vi "Ref_Num_Generate_Report_NEW.vi"(0 "LowCapMode?":refnum<vi>, 1 "Test Part":refnum<vi>, 2 "Test Voltages(V)":refnum<vi>, 3 "T.V. True":refnum<vi>, 4 "Stop":refnum<vi>, 5 "error in (no error)":errorcluster, 6 "Array":refnum<vi>, 7 "Chart Voltage Generation Method":refnum<vi>, 8 "XY Graph NEW":refnum<vi>, 10 "CapTest?":refnum<vi>, 11 "Polarity for Max Voltage":refnum<vi>, 12 "Test Voltages Chosen":refnum<vi>, 13 "Capacitance(pF)":refnum<vi>, 14 "Min Voltage":refnum<vi>, 15 "Max Voltage":refnum<vi>, 17 "Status : Running":refnum<vi>, 18 "Next Part":refnum<vi>) -> (19 "error out":errorcluster)   [LabVIEW 2020]
uses:
  Global 1.vi
  <vilib>/Utility/file.llb/Write Delimited Spreadsheet (DBL).vi
  <vilib>/Utility/file.llb/Write Delimited Spreadsheet (string).vi
panel:
  out "error out 2":errorcluster
  in  "Test Voltages TRUE":bool
  in  "Test Voltages Results Temp Array":dbl[](array[numeric]) format="%_6g"
  out "Status : Running+-":bool
  in  "Test Voltages (in)":dbl[](array[numeric])=[0.0, 0.1, 0.2, 0.3, 0.4, 0.5, 0.7, 1.0, 2.0, 3.0, 4.0, 5.0, 7.0, 10.0, 20.0, 30.0, 40.0, 50.0, 70.0, 100.0, 200.0]
  in  "Capacitance Results Temp Array":dbl[](array[numeric]) format="%_10g"
  in  "Default":i32=1
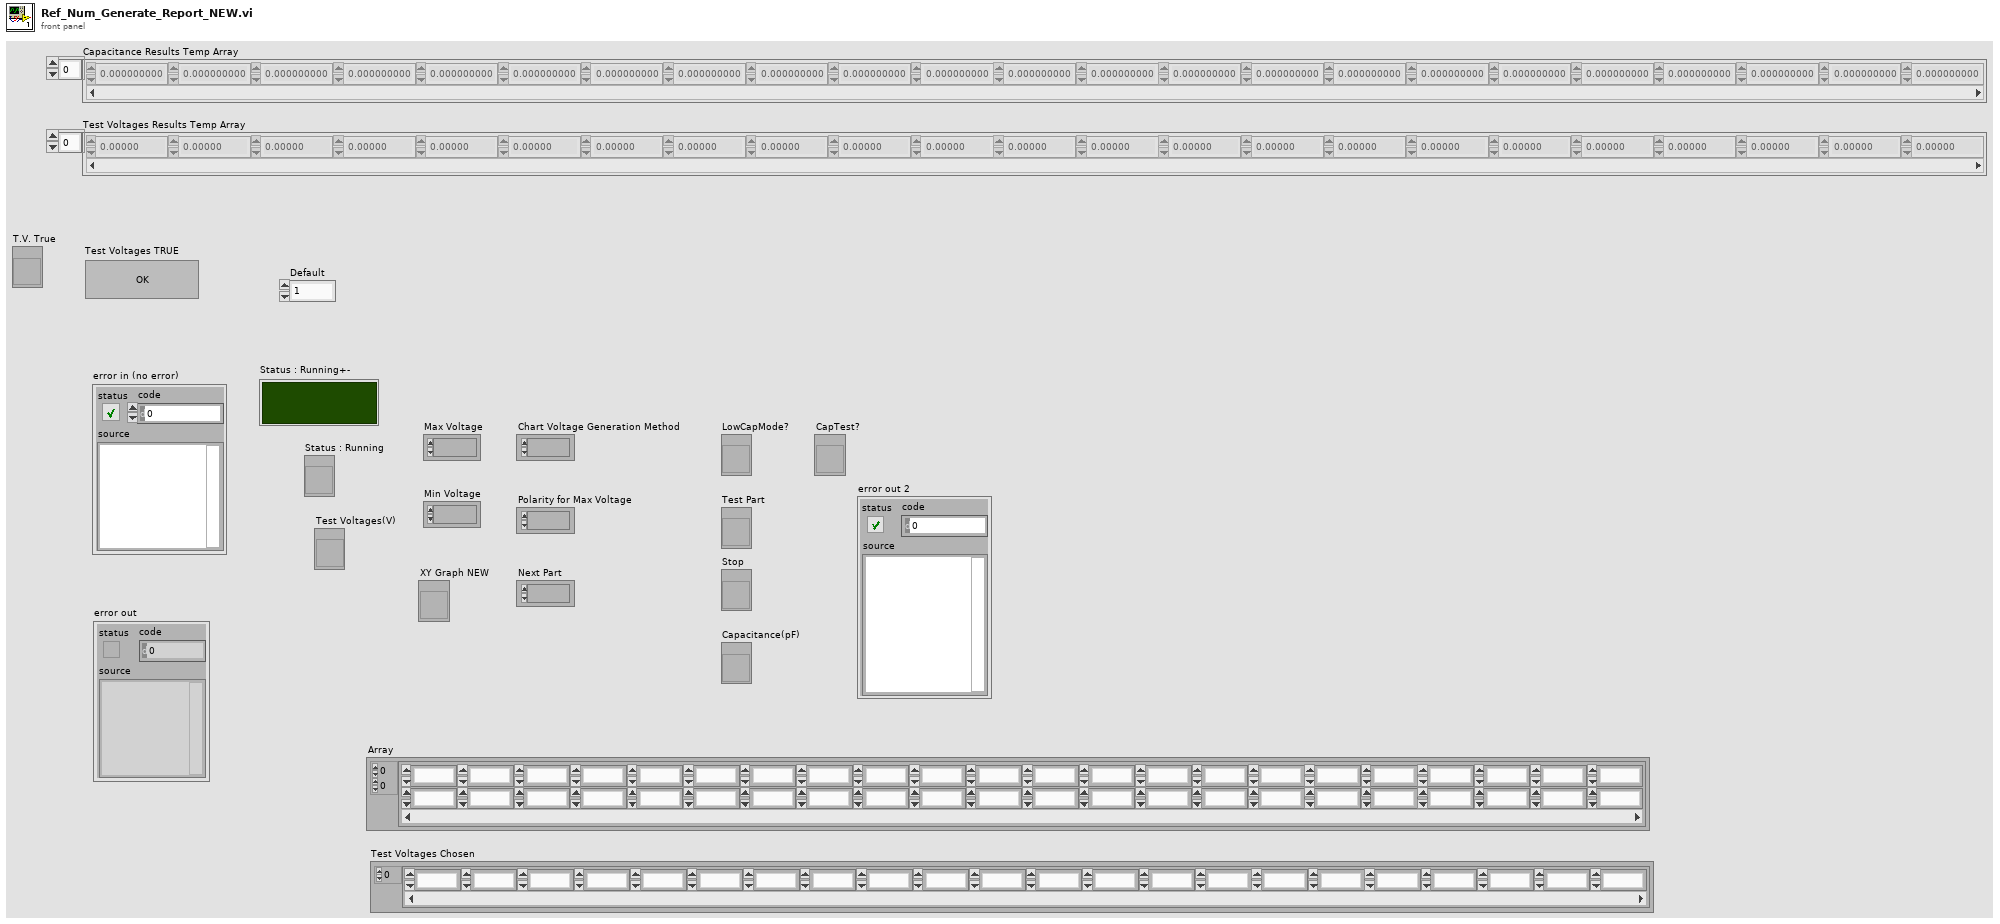
[diagram p1: front panel]
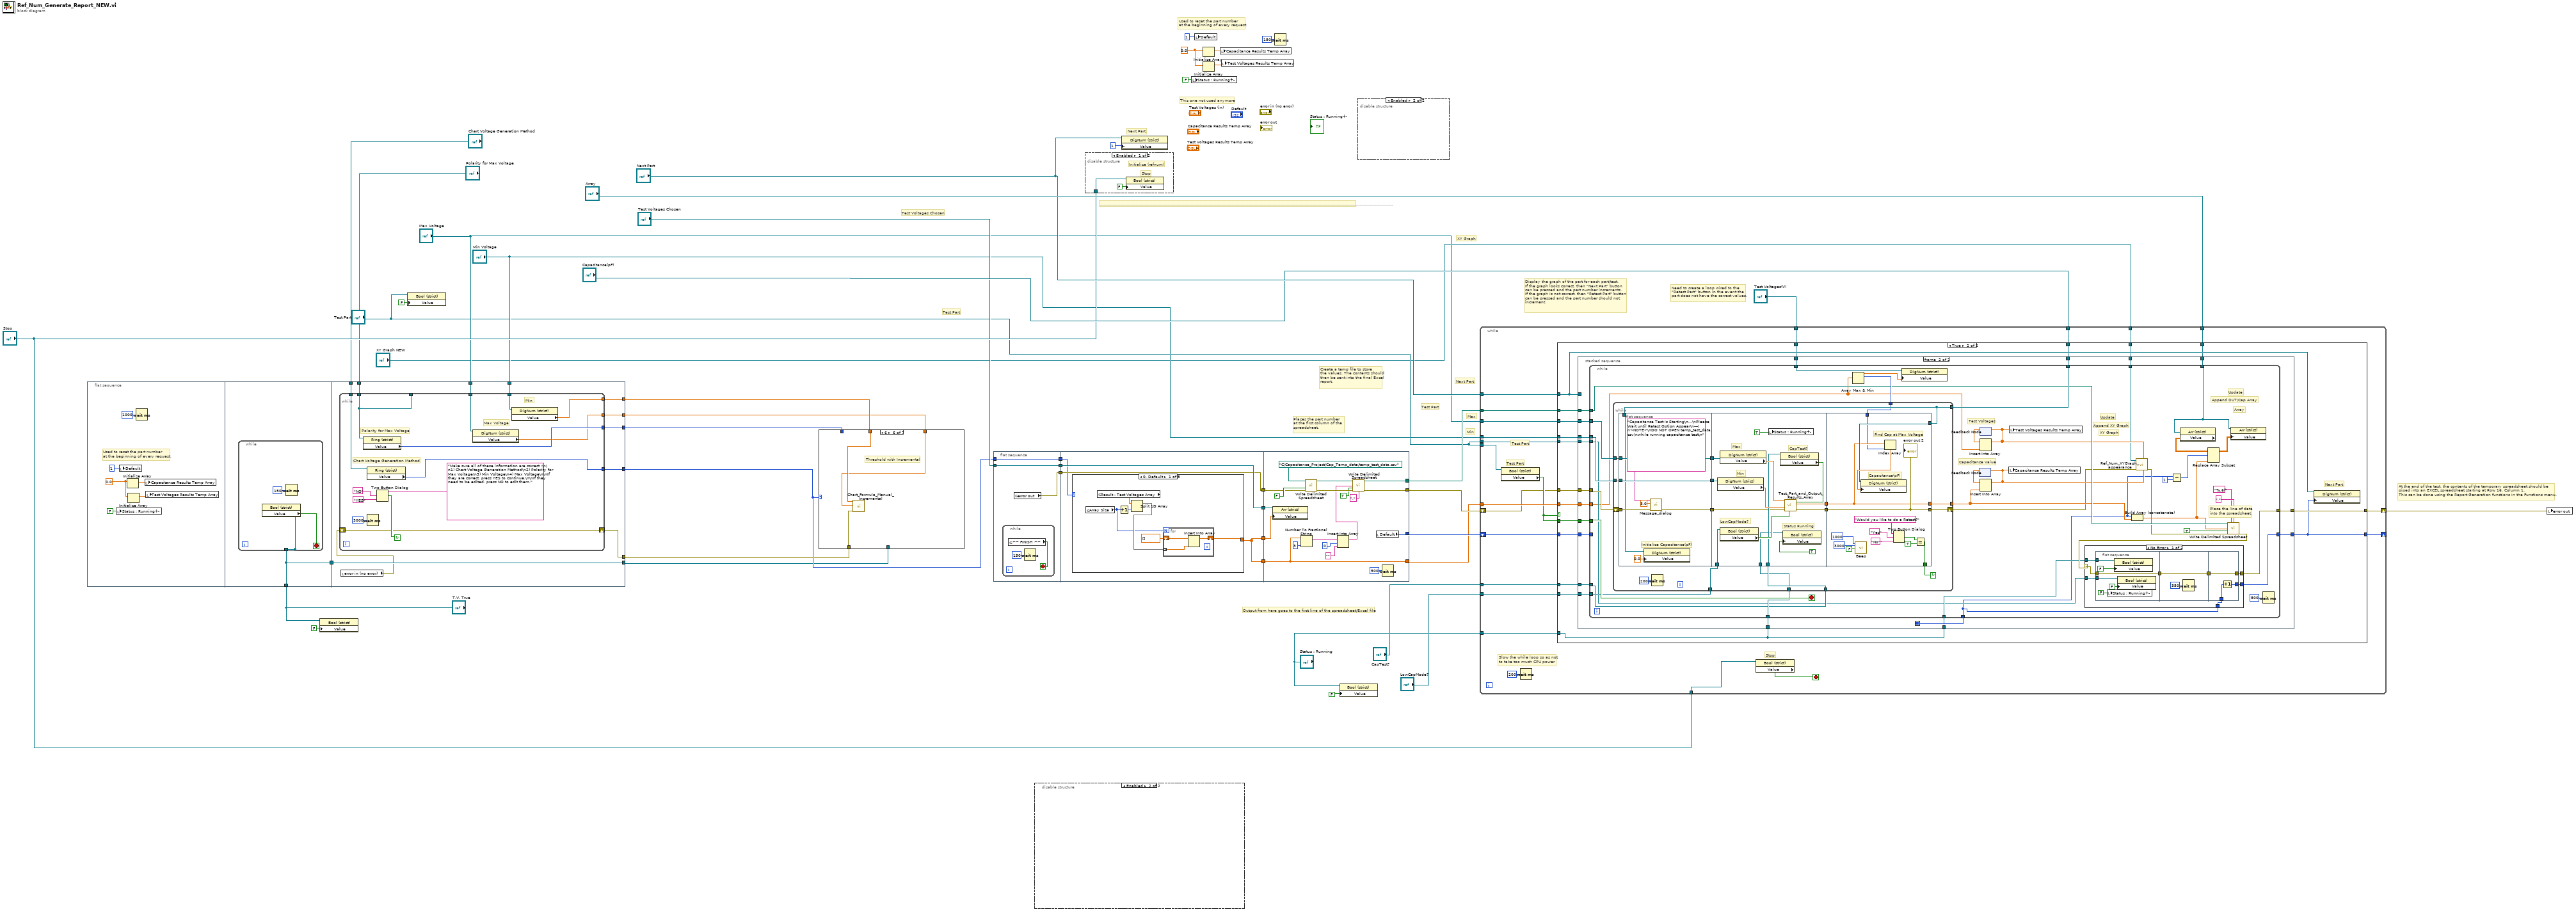
[diagram p0: block diagram]
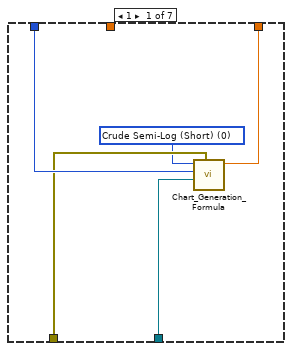
[diagram p2: hidden frame]
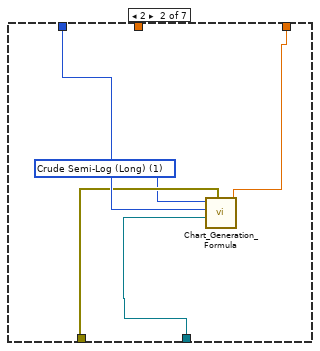
[diagram p3: hidden frame]
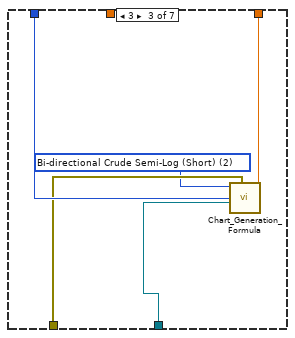
[diagram p4: hidden frame]
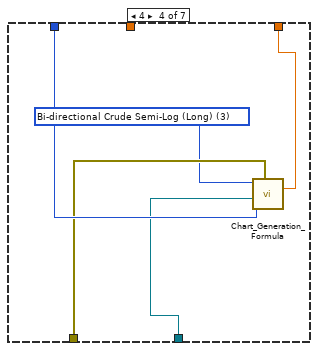
[diagram p5: hidden frame]
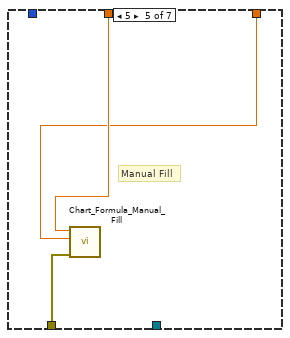
[diagram p6: hidden frame]
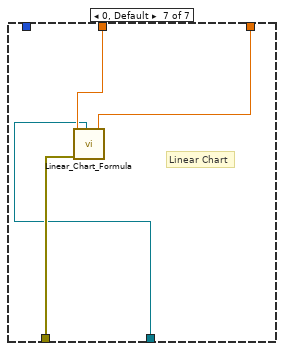
[diagram p7: hidden frame]
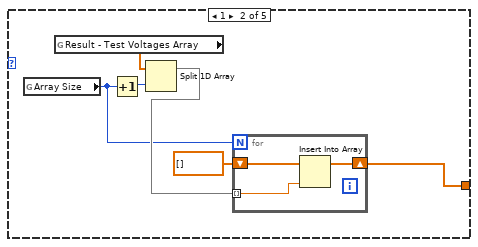
[diagram p8: hidden frame]
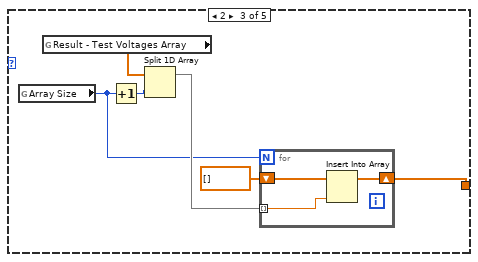
[diagram p9: hidden frame]
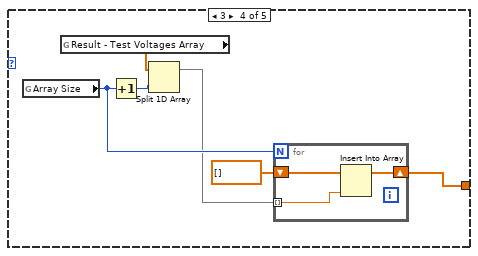
[diagram p10: hidden frame]
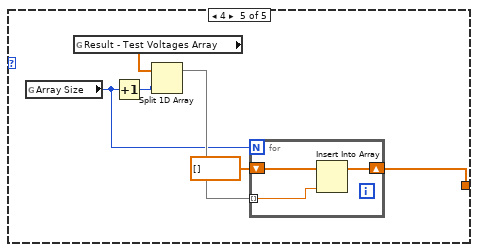
[diagram p11: hidden frame]
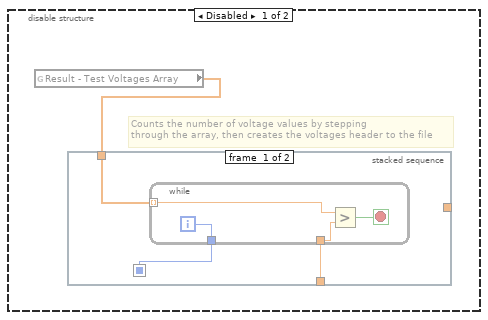
[diagram p13: hidden frame]
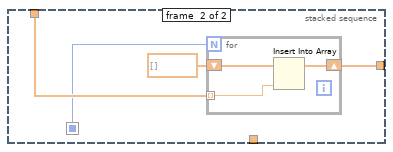
[diagram p14: hidden frame]
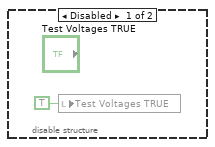
[diagram p15: hidden frame]
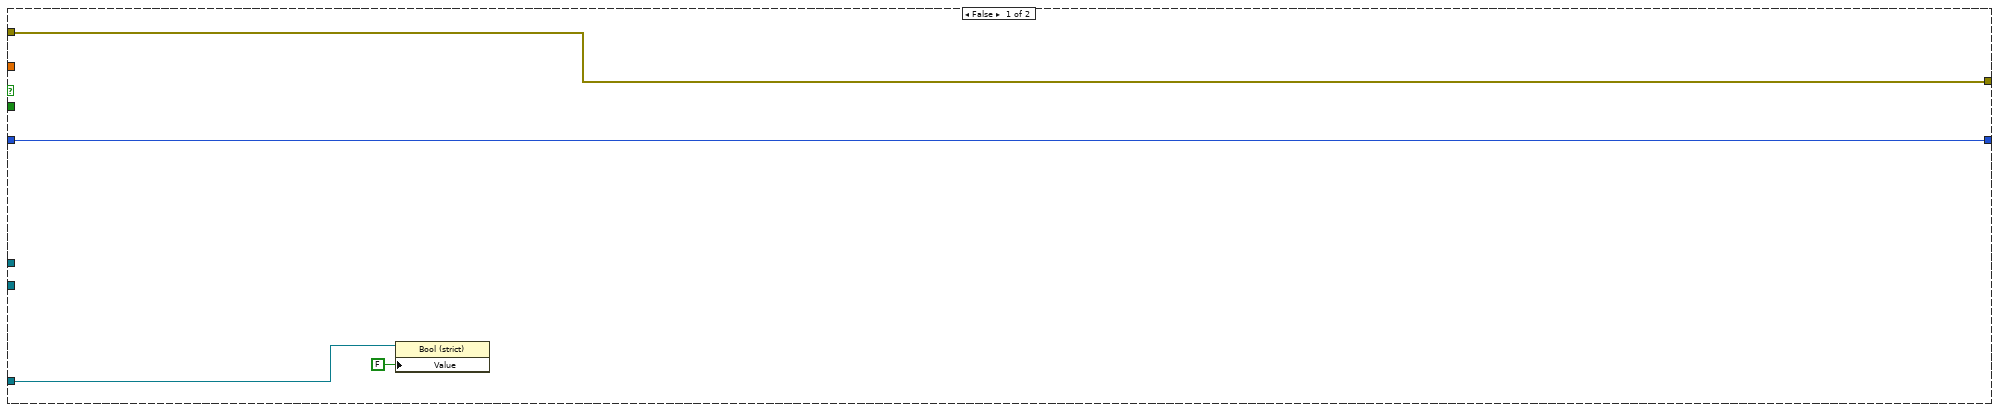
[diagram p16: hidden frame]
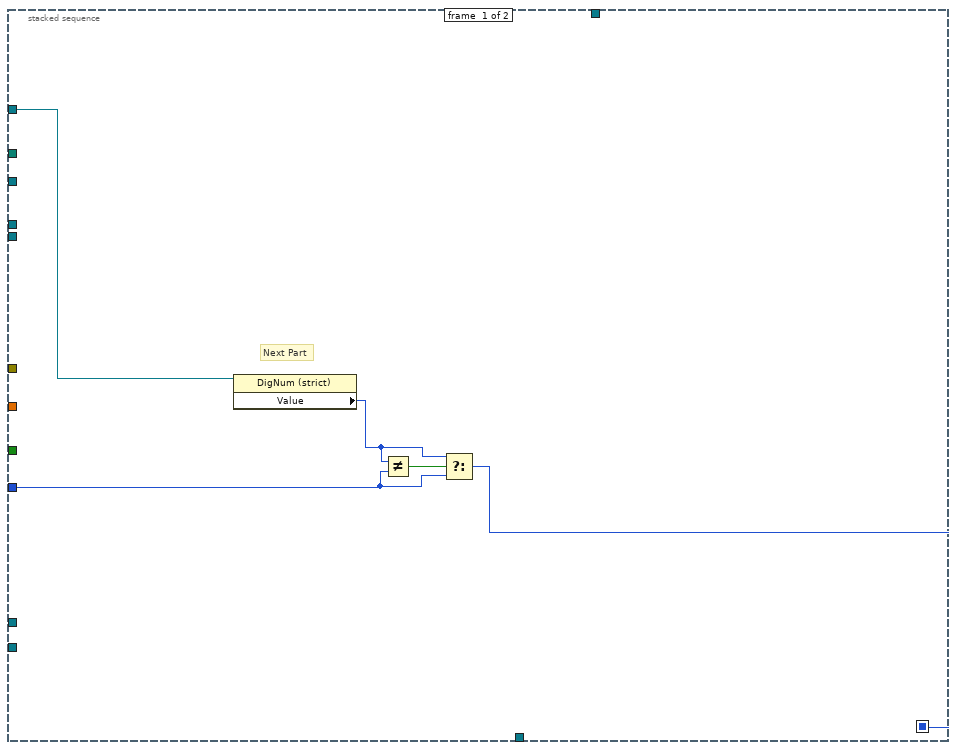
[diagram p17: hidden frame]
diagram:
  w6 = 0.0 ("element")
  # "Places the part number\nat the first column of the \nspreadsheet."
  # "Used to reset the part number\nat the beginning of every request."
  # "XY Graph"
  # "Need to create a loop wired to the \n\"Retest Part\" button in the event the \npart does not have the correct values."
  # "Display the graph of the part for each part/test.\nIf the graph looks correct, then \"Next Part\" button\ncan be pressed and the part number increments.\nIf the graph is not correct, then \"Retest Part\" button\ncan be pressed and the part number should not\nincrement."
  # "This one not used anymore"
  # "Test Part"
  # "Test Part"
  # "Min"
  # "Max"
  # "Test Voltages Chosen"
  # "....................................................................................................................................................................................................................................."
  # "Next Part"
  # "Next Part"
  # "At the end of the test, the contents of the temporary spreadsheet should be\npiped into an EXCEL spreadsheet starting at Row 16, Column 1. \nThis can be done using the Report Generation functions in the Functions menu."
  # "Create a temp file to store\nthe values. The contents should\nthen be sent into the final Excel\nreport."
  # "Output from here goes to the first line of the spreadsheet/Excel file"
  n1 = flat-sequence {
    tunnel: "T.V. True" -> [w52]
    tunnel: [w52] -> w1
    tunnel: "Chart Voltage Generation Method" -> [w66]
    tunnel: "Polarity for Max Voltage" -> [w65]
    tunnel: "Max Voltage" -> [w64]
    tunnel: "Min Voltage" -> [w63]
    tunnel: w1 -> [w58]
    tunnel: [w62] -> w21
    tunnel: [w61] -> w20
    tunnel: [w60] -> w19
    tunnel: [w59] -> w18
    tunnel: [w56] -> w17
    tunnel: [w58] -> w2
    frame #0 {
      w48 = 0.0 ("element")
      # "Used to reset the part number\nat the beginning of every request."
      n2 = local write "Status : Running+-"(FALSE ("Status : Running+-")) -> ()
      n3 = local write "Default"(1 ("New Part Number")) -> ()
      n4 = Initialize Array(w48) -> (w49:dbl[])  [unwired: 1 in]
      n5 = Initialize Array(w48) -> (w50:dbl[])  [unwired: 1 in]
      n6 = Wait (ms)(milliseconds to wait=u32 1000) -> ()  [unwired: 1 out]
      n7 = local write "Capacitance Results Temp Array"(w49) -> ()
      n8 = local write "Test Voltages Results Temp Array"(w50) -> ()
    }
    frame #1 {
      n9 = while {
        tunnel: w52 -> [w54]
        tunnel: [w54] -> _
        stop <- w55 stop-if-true
        n10 = property class="Bool (strict)"(reference=w54) -> ("Value"=w55:bool)  [unwired: 1 in, 2 out]
        n11 = Wait (ms)(milliseconds to wait=u32 150) -> ()  [unwired: 1 out]
      }
    }
    frame #2 {
      n12 = local read "error in (no error)"() -> (w57:errorcluster)
      n13 = while {
        tunnel: w66 -> [w75]
        tunnel: [w74] -> w59
        tunnel: w65 -> [w68]
        tunnel: [w73] -> w60
        tunnel: w64 -> [w72]
        tunnel: [w71] -> w61
        tunnel: w63 -> [w70]
        tunnel: [w69] -> w62
        tunnel: [w68] -> _
        shift-right: [w67] -> w56
        shift-left: w57 -> [w67]
        stop <- w77 continue-if-true
        # "Min"
        # "Max Voltage"
        # "Polarity for Max Voltage"
        # "Chart Voltage Generation Method"
        n14 = property class="Ring (strict)"(reference=w68) -> ("Value"=w73:u16)  [unwired: 1 in, 2 out]
        n15 = Wait (ms)(milliseconds to wait=u32 3000) -> ()  [unwired: 1 out]
        n16 = property class="Ring (strict)"(reference=w75) -> ("Value"=w74:u16)  [unwired: 1 in, 2 out]
        n17 = Two Button Dialog(message="Make sure all of these information are correct :\n\n1) Chart Voltage Generation Method\n2) Polarity for Max Voltage\n3) Min Voltage\n4) Max Voltage\n\nIf they are correct, press YES to continue.\n\nIf they need to be edited, press NO to edit them.", 1:"YES" ("Right Button Text (\"Cancel\")"), 2:"NO" ("Left Button Text (\"Yes\")")) -> (T button?=w77:bool)
        n18 = property class="DigNum (strict)"(reference=w72) -> ("Value"=w71:dbl)  [unwired: 1 in, 2 out]
        n19 = property class="DigNum (strict)"(reference=w70) -> ("Value"=w69:dbl)  [unwired: 1 in, 2 out]
      }
    }
  }
  n20 = property class="Bool (strict)"(reference="T.V. True", "Value"=FALSE) -> ()  [unwired: 1 in, 2 out]
  n21 = property class="Bool (strict)"(reference="Test Part", "Value"=FALSE) -> ()  [unwired: 1 in, 2 out]
  n22 = case shown="6" w18 {
    tunnel: w19 -> [w85 w90 w95 w100 _ _ _]
    tunnel: w20 -> [w84 w89 w94 w99 w101 w104 w109]
    tunnel: w2 -> [w83 w88 w93 w98 _ _ w107]
    tunnel: w17 -> [w82 w87 w92 w97 w103 w106 w110]
    tunnel: w21 -> [_ _ _ _ w102 w105 w108]
    frame 1 {
      w81 = u16 0 items=[" Crude Semi-Log (Short)", "Crude Semi-Log (Long)", "Bi-directional Crude Semi-Log (Short)", "Bi-directional Crude Semi-Log (Long)"] ("Type of Chart")
      n23 = call "Chart_Generation_Formula.vi"("Max Voltage"=w84, "error in (no error)"=w82, "CGF_Input"=w83, "Polarity for Max Voltage"=w85, "Type of Chart"=w81) -> ()  [unwired: 4 in, 3 out]
    }
    frame 2 {
      w86 = u16 1 items=[" Crude Semi-Log (Short)", "Crude Semi-Log (Long)", "Bi-directional Crude Semi-Log (Short)", "Bi-directional Crude Semi-Log (Long)"] ("Type of Chart")
      n24 = call "Chart_Generation_Formula.vi"("Max Voltage"=w89, "error in (no error)"=w87, "CGF_Input"=w88, "Polarity for Max Voltage"=w90, "Type of Chart"=w86) -> ()  [unwired: 4 in, 3 out]
    }
    frame 3 {
      w91 = u16 2 items=[" Crude Semi-Log (Short)", "Crude Semi-Log (Long)", "Bi-directional Crude Semi-Log (Short)", "Bi-directional Crude Semi-Log (Long)"] ("Type of Chart")
      n25 = call "Chart_Generation_Formula.vi"("Max Voltage"=w94, "error in (no error)"=w92, "CGF_Input"=w93, "Polarity for Max Voltage"=w95, "Type of Chart"=w91) -> ()  [unwired: 4 in, 3 out]
    }
    frame 4 {
      w96 = u16 3 items=[" Crude Semi-Log (Short)", "Crude Semi-Log (Long)", "Bi-directional Crude Semi-Log (Short)", "Bi-directional Crude Semi-Log (Long)"] ("Type of Chart")
      n26 = call "Chart_Generation_Formula.vi"("Max Voltage"=w99, "error in (no error)"=w97, "CGF_Input"=w98, "Polarity for Max Voltage"=w100, "Type of Chart"=w96) -> ()  [unwired: 4 in, 3 out]
    }
    frame 5 {
      # "Manual Fill"
      n27 = call "Chart_Formula_Manual_Fill.vi"("error in (no error)"=w103, "Max Voltage"=w101, "Min Voltage"=w102) -> ()  [unwired: 9 in]
    }
    frame 6 {
      # "Threshold with Incremental"
      n28 = call "Chart_Formula_Manual_Incremental.vi"("error in (no error)"=w106, "Max Voltage"=w104, "Min Voltage"=w105) -> ()  [unwired: 8 in]
    }
    frame 0, Default {
      # "Linear Chart"
      n29 = call "Linear_Chart_Formula.vi"("Max Voltage"=w109, "Start"=w107, "error in (no error)"=w110, "Min Voltage"=w108) -> ()  [unwired: 7 in, 1 out]
    }
  }
  n30 = flat-sequence {
    tunnel: w18 -> [w112]
    tunnel: "Test Voltages Chosen" -> [w113]
    tunnel: [w113] -> w25
    tunnel: [w112] -> w24
    tunnel: [w111] -> w22
    tunnel: [w118] -> w30
    tunnel: [w116] -> w29
    tunnel: [w119] -> w28
    tunnel: [w118] -> w27
    tunnel: w25 -> [w119]
    tunnel: w24 -> [w117]
    tunnel: w22 -> [w116]
    tunnel: w30 -> [w166]
    tunnel: w29 -> [w169]
    tunnel: w28 -> [w168]
    tunnel: w27 -> [w167]
    tunnel: [w179] -> w45
    tunnel: [w176] -> w44
    tunnel: [w174] -> w35
    tunnel: [w166] -> w26
    frame #0 {
      n31 = while {
        stop <- w115 stop-if-true
        n32 = global read "Global 1.vi" "~~ FINISH ~~"() -> (w115:bool)
        n33 = Wait (ms)(milliseconds to wait=u32 150) -> ()  [unwired: 1 out]
      }
      n34 = global read "Global 1.vi" "error out"() -> (w111:errorcluster)
    }
    frame #1 {
      n35 = case shown="0, Default" w117 {
        tunnel: [w120 w129 w138 w147 w156] -> w118
        frame 0, Default {
          n36 = global read "Global 1.vi" "Array Size"() -> (w122:i32)
          n37 = global read "Global 1.vi" "Result - Test Voltages Array"() -> (w125:dbl[])
          n38 = Increment(x=w122) -> (x+1=w124:i32)
          n39 = Split 1D Array(array=w125, index=w124) -> (first subarray=w123:dbl[])  [unwired: 1 out]
          n40 = for {
            N: w122 -> [_]
            tunnel: w123 -> [w128] mode=indexing
            shift-right: [w126] -> w120
            shift-left: dbl[] [] -> [w127]
            n41 = Insert Into Array(array=w127, new element=w128) -> (w126:dbl[])  [unwired: 1 in]
          }
        }
        frame 1 {
          n42 = global read "Global 1.vi" "Array Size"() -> (w130:i32)
          n43 = global read "Global 1.vi" "Result - Test Voltages Array"() -> (w134:dbl[])
          n44 = Increment(x=w130) -> (x+1=w133:i32)
          n45 = Split 1D Array(array=w134, index=w133) -> (first subarray=w131:dbl[])  [unwired: 1 out]
          n46 = for {
            N: w130 -> [_]
            tunnel: w131 -> [w137] mode=indexing
            shift-right: [w135] -> w129
            shift-left: dbl[] [] -> [w136]
            n47 = Insert Into Array(array=w136, new element=w137) -> (w135:dbl[])  [unwired: 1 in]
          }
        }
        frame 2 {
          n48 = global read "Global 1.vi" "Array Size"() -> (w139:i32)
          n49 = global read "Global 1.vi" "Result - Test Voltages Array"() -> (w142:dbl[])
          n50 = Increment(x=w139) -> (x+1=w143:i32)
          n51 = Split 1D Array(array=w142, index=w143) -> (first subarray=w140:dbl[])  [unwired: 1 out]
          n52 = for {
            N: w139 -> [_]
            tunnel: w140 -> [w146] mode=indexing
            shift-right: [w144] -> w138
            shift-left: dbl[] [] -> [w145]
            n53 = Insert Into Array(array=w145, new element=w146) -> (w144:dbl[])  [unwired: 1 in]
          }
        }
        frame 3 {
          n54 = global read "Global 1.vi" "Array Size"() -> (w149:i32)
          n55 = global read "Global 1.vi" "Result - Test Voltages Array"() -> (w151:dbl[])
          n56 = Increment(x=w149) -> (x+1=w152:i32)
          n57 = Split 1D Array(array=w151, index=w152) -> (first subarray=w148:dbl[])  [unwired: 1 out]
          n58 = for {
            N: w149 -> [_]
            tunnel: w148 -> [w155] mode=indexing
            shift-right: [w153] -> w147
            shift-left: dbl[] [] -> [w154]
            n59 = Insert Into Array(array=w154, new element=w155) -> (w153:dbl[])  [unwired: 1 in]
          }
        }
        frame 4 {
          n60 = global read "Global 1.vi" "Array Size"() -> (w157:i32)
          n61 = global read "Global 1.vi" "Result - Test Voltages Array"() -> (w160:dbl[])
          n62 = Increment(x=w157) -> (x+1=w161:i32)
          n63 = Split 1D Array(array=w160, index=w161) -> (first subarray=w158:dbl[])  [unwired: 1 out]
          n64 = for {
            N: w157 -> [_]
            tunnel: w158 -> [w164] mode=indexing
            shift-right: [w162] -> w156
            shift-left: dbl[] [] -> [w163]
            n65 = Insert Into Array(array=w163, new element=w164) -> (w162:dbl[])  [unwired: 1 in]
          }
        }
      }
    }
    frame #2 {
      n66 = property class="Arr (strict)"(reference=w168, "Value"=w167) -> ()  [unwired: 1 in, 2 out]
      n67 = Number To Fractional String(number=w166, precision (6)=i16 3) -> (F-format string=w182:string[])  [unwired: 2 in]
      n68 = call-poly <vilib>:"Write Delimited Spreadsheet.vi"("file path (dialog if empty)"=path "C:/Capacitance_Project/Cap_Temp_data/temp_test_data.csv", "append to file? (new file:F)"=FALSE, "error in (no error)"=w169) -> ("new file path (Not A Path if cancelled)"=w177:path, "error out"=w175:errorcluster)  [unwired: 11 in]
      n69 = Insert Into Array(array=w182, index=0, new element="" ("new element/subarray")) -> (w173:string[])
      n70 = call-poly <vilib>:"Write Delimited Spreadsheet.vi"("file path (dialog if empty)"=w177, "1D data"=w173, "append to file? (new file:F)"=TRUE, "error in (no error)"=w175, "delimiter (\\t)"="," ("delimiter (\\t)")) -> ("new file path (Not A Path if cancelled)"=w176:path, "error out"=w174:errorcluster)  [unwired: 9 in]
      n71 = local read "Default"() -> (w179:i32)
      n72 = Wait (ms)(milliseconds to wait=u32 500) -> ()  [unwired: 1 out]
    }
  }
  n73 = disable-structure shown="Enabled" {
    frame Disabled {
      # "Counts the number of voltage values by stepping\nthrough the array, then creates the voltages header to the file"
      n74 = global read "Global 1.vi" "Result - Test Voltages Array"() -> (w184:dbl[])
      n75 = stacked-sequence {
        seq-local: [w186 _] -> [_ w193]
        tunnel: w184 -> [w187 w194]
        tunnel: [_ w195] -> _
        tunnel: _ -> [w185 _]
        frame #0 {
          n76 = while {
            tunnel: w187 -> [w190] mode=indexing
            tunnel: [w189] -> w186
            tunnel: w185 -> [w188]
            i -> [w189]
            stop <- w191 stop-if-true
            n77 = Greater?(x=w190, y=w188) -> (0:w191:bool)
          }
        }
        frame #1 {
          n78 = for {
            N: w193 -> [_]
            tunnel: w194 -> [w198] mode=indexing
            shift-right: [w196] -> w195
            shift-left: dbl[] [] -> [w197]
            n79 = Insert Into Array(array=w197, new element=w198) -> (w196:dbl[])  [unwired: 1 in]
          }
        }
      }
    }
    frame Enabled {
    }
  }
  n80 = disable-structure shown="Enabled" {
    disable-tunnel: "Stop" -> [w199 _]
    frame Enabled {
      # "Stop"
      # "Initialize (refnum)"
      n81 = property class="Bool (strict)"(reference=w199, "Value"=FALSE) -> ()  [unwired: 1 in, 2 out]
    }
    frame Disabled {
    }
  }
  n82 = property class="DigNum (strict)"(reference="Next Part", "Value"=1) -> ()  [unwired: 1 in, 2 out]
  n83 = local write "Status : Running+-"(FALSE ("Status : Running+-")) -> ()
  n84 = local write "Default"(1 ("New Part Number")) -> ()
  n85 = Initialize Array(w6) -> (w5:dbl[])  [unwired: 1 in]
  n86 = Initialize Array(w6) -> (w4:dbl[])  [unwired: 1 in]
  n87 = local write "Capacitance Results Temp Array"(w5) -> ()
  n88 = local write "Test Voltages Results Temp Array"(w4) -> ()
  n89 = Wait (ms)(milliseconds to wait=u32 150) -> ()  [unwired: 1 out]
  n90 = property class="Bool (strict)"(reference="Status : Running", "Value"=FALSE) -> ()  [unwired: 1 in, 2 out]
  n91 = disable-structure shown="Enabled" {
    frame Disabled {
      n92 = local write "Test Voltages TRUE"(TRUE ("Test Voltages TRUE")) -> ()
    }
    frame Enabled {
    }
  }
  n93 = while {
    tunnel: w26 -> [w223]
    shift-right: [w220] -> _
    shift-left: w45 -> [w221]
    tunnel: w44 -> [w218]
    tunnel: "Next Part" -> [w217]
    tunnel: "Array" -> [w216]
    tunnel: "Max Voltage" -> [w215]
    tunnel: "Min Voltage" -> [w214]
    tunnel: "Capacitance(pF)" -> [w213]
    tunnel: "Test Part" -> [w212]
    tunnel: "Test Part" -> [w210]
    tunnel: "Stop" -> [w209]
    tunnel: "XY Graph NEW" -> [w207]
    tunnel: "Status : Running" -> [w206]
    tunnel: "CapTest?" -> [w205]
    shift-right: [w219] -> w38
    shift-left: w35 -> [w204]
    tunnel: "Test Voltages(V)" -> [w203]
    tunnel: "LowCapMode?" -> [w202]
    stop <- w208 stop-if-true
    # "Stop"
    # "Test Part"
    # "Test Part"
    # "Slow the while loop so as not\nto take too much CPU power"
    n94 = property class="Bool (strict)"(reference=w212) -> ("Value"=w211:bool)  [unwired: 1 in, 2 out]
    n95 = Wait (ms)(milliseconds to wait=u32 200) -> ()  [unwired: 1 out]
    n96 = case shown="True" w211 {
      tunnel: w223 -> [_ w244]
      tunnel: w211 -> [_ w245]
      tunnel: w221 -> [w227 w241]
      tunnel: [w227 w239] -> w220
      tunnel: [w226 w243] -> w219
      tunnel: w204 -> [w226 w242]
      tunnel: w218 -> [_ w240]
      tunnel: w217 -> [_ w238]
      tunnel: w216 -> [_ w237]
      tunnel: w215 -> [_ w236]
      tunnel: w214 -> [_ w235]
      tunnel: w213 -> [_ w234]
      tunnel: w210 -> [_ w233]
      tunnel: w207 -> [_ w232]
      tunnel: w206 -> [w224 w231]
      tunnel: w205 -> [_ w230]
      tunnel: w203 -> [_ w229]
      tunnel: w202 -> [_ w228]
      frame False {
        n97 = property class="Bool (strict)"(reference=w224, "Value"=FALSE) -> ()  [unwired: 1 in, 2 out]
      }
      frame True {
        # "Next Part"
        n98 = stacked-sequence {
          seq-local: [w249 _] -> [_ w264]
          tunnel: [_ w269] -> w239
          tunnel: w245 -> [_ w268]
          tunnel: w244 -> [_ w267]
          tunnel: [_ w254] -> w243
          tunnel: w242 -> [_ w266]
          tunnel: w241 -> [w248 w265]
          tunnel: w240 -> [_ w263]
          tunnel: w238 -> [w247 _]
          tunnel: w237 -> [_ w262]
          tunnel: w236 -> [_ w261]
          tunnel: w235 -> [_ w260]
          tunnel: w234 -> [_ w259]
          tunnel: w233 -> [_ w258]
          tunnel: w232 -> [_ w257]
          tunnel: w231 -> [_ w256]
          tunnel: w231 -> [_ w255]
          tunnel: w230 -> [_ w253]
          tunnel: w229 -> [_ w252]
          tunnel: w228 -> [_ w251]
          frame #0 {
            # "Next Part"
            n99 = property class="DigNum (strict)"(reference=w247) -> ("Value"=w246:i32)  [unwired: 1 in, 2 out]
            n100 = Not Equal?(x=w246, y=w248) -> (x != y?=w250:bool)
            n101 = Select(t=w246, s=w250, f=w248) -> (s? t:f=w249:i32)
          }
          frame #1 {
            n102 = while {
              tunnel: w267 -> [w283]
              tunnel: w268 -> [w303]
              tunnel: w265 -> [_]
              tunnel: [w296] -> w269
              tunnel: w266 -> [w302]
              tunnel: w264 -> [w272]
              tunnel: w263 -> [w286]
              tunnel: w262 -> [w274]
              tunnel: w261 -> [w301]
              tunnel: w260 -> [w300]
              tunnel: w259 -> [w299]
              tunnel: w258 -> [w284]
              tunnel: w257 -> [w277]
              tunnel: w256 -> [w295]
              tunnel: w255 -> [w285]
              tunnel: [w293] -> w254
              tunnel: w253 -> [w287]
              tunnel: w252 -> [w291]
              tunnel: w251 -> [w289]
              stop <- w303 stop-if-true
              # "Append XY Graph"
              # "Update"
              # "Update"
              # "Append DUT/Cap Array"
              # "Capacitance Value"
              # "Test Voltages"
              # "XY Graph"
              # "Array"
              # "Place the line of data\ninto the spreadsheet."
              n103 = Array Max & Min(array=w283) -> (max value=w290:dbl, max index (indices)=w292:i32)  [unwired: 2 out]
              n104 = while {
                shift-right: [w341] -> w279
                shift-left: w302 -> [w342]
                tunnel: [w340] -> w282
                tunnel: w301 -> [w338]
                tunnel: w300 -> [w337]
                tunnel: w299 -> [w334]
                tunnel: w295 -> [w330]
                tunnel: w287 -> [w331]
                tunnel: w292 -> [w333]
                tunnel: w289 -> [w329]
                stop <- w332 continue-if-true
                n105 = flat-sequence {
                  tunnel: w337 -> [w349]
                  tunnel: w338 -> [w350]
                  tunnel: w342 -> [w346]
                  tunnel: [w345] -> w328
                  tunnel: [w350] -> w327
                  tunnel: [w349] -> w326
                  tunnel: w334 -> [w348]
                  tunnel: [w353] -> w336
                  tunnel: [w352] -> w335
                  tunnel: w331 -> [w360]
                  tunnel: w330 -> [w359]
                  tunnel: w329 -> [w351]
                  tunnel: w327 -> [w355]
                  tunnel: w326 -> [w356]
                  tunnel: w328 -> [w354]
                  tunnel: [w372] -> w340
                  tunnel: [w374] -> w341
                  tunnel: w336 -> [w374]
                  tunnel: w335 -> [w372]
                  tunnel: w334 -> [w373]
                  tunnel: w333 -> [w368]
                  tunnel: [w369] -> w332
                  frame #0 {
                    # "Initialize Capacitance(pF)"
                    n106 = property class="DigNum (strict)"(reference=w348, "Value"=0.0) -> ()  [unwired: 1 in, 2 out]
                    n107 = call "Message_dialog.vi"("error in (no error)"=w346, "set delay"=3.0, "String"="Capacitance Test is Starting\n...\nPlease Wait until Retest Option Appear\n---\n<NOTE>\nDO NOT OPEN temp_test_data.csv\nwhile running capacitance test\n" ("message")) -> ("error out"=w345:errorcluster)  [unwired: 8 in]
                  }
                  frame #1 {
                    # "LowCapMode?"
                    # "Status Running"
                    # "CapTest?"
                    # "Min"
                    # "Max"
                    n108 = property class="DigNum (strict)"(reference=w356) -> ("Value"=w362:dbl)  [unwired: 1 in, 2 out]
                    n109 = property class="DigNum (strict)"(reference=w355) -> ("Value"=w361:dbl)  [unwired: 1 in, 2 out]
                    n110 = property class="Bool (strict)"(reference=w351) -> ("Value"=w364:bool)  [unwired: 1 in, 2 out]
                    n111 = local write "Status : Running+-"(TRUE ("Status : Running+-")) -> ()
                    n112 = property class="Bool (strict)"(reference=w360) -> ("Value"=w363:bool)  [unwired: 1 in, 2 out]
                    n113 = property class="Bool (strict)"(reference=w359, "Value"=TRUE) -> ()  [unwired: 1 in, 2 out]
                    n114 = call "Test_Part_and_Output_Results_Array.vi"("CapTest?"=w363, "LowCapMode?"=w364, "error in"=w354, "Min Voltage"=w362, "Max Voltage"=w361) -> ("error out"=w353:errorcluster, "Capacitance Results Array"=w352:dbl[])  [unwired: 3 in, 2 out]
                  }
                  frame #2 {
                    # "Find Cap at Max Voltage"
                    # "Capacitance(pF)"
                    n115 = call <vilib>:"Beep.vi"("use system alert? (T)"=FALSE, "duration (msec)"=u32 3000, "frequency (Hz)"=u32 1000) -> ()  [unwired: 9 in]
                    n116 = Index Array(array=w372, index=w368) -> (element=w375:dbl)
                    n117 = property class="DigNum (strict)"(reference=w373, "Value"=w375) -> ()  [unwired: 1 in, 2 out]
                    n118 = Two Button Dialog(message="Would you like to do a Retest?", 1:"No" ("Right Button Text (\"Cancel\")"), 2:"Yes" ("Left Button Text (\"Yes\")")) -> (T button?=w370:bool)
                    n119 = Equal?(x=w370, y=TRUE) -> (x = y?=w369:bool)
                    "error out 2" <- w374
                  }
                }
                n120 = Wait (ms)(milliseconds to wait=u32 200) -> ()  [unwired: 1 out]
              }
              n121 = property class="DigNum (strict)"(reference=w291, "Value"=w290) -> ()  [unwired: 1 in, 2 out]
              n122 = feedback #1() -> (w298:dbl[])  [unwired: 1 in]
              n123 = feedback #2() -> (w297:dbl[])  [unwired: 1 in]
              n124 = Insert Into Array(array=w297, new element=w283) -> (w281:dbl[])  [unwired: 1 in]
              n125 = feedback-in #2(w281) -> ()
              n126 = Insert Into Array(array=w298, new element=w282) -> (w280:dbl[])  [unwired: 1 in]
              n127 = feedback-in #1(w280) -> ()
              n128 = local write "Capacitance Results Temp Array"(w280) -> ()
              n129 = local write "Test Voltages Results Temp Array"(w281) -> ()
              n130 = Build Array (concatenate)(w272, w282) -> (w270:dbl[])
              n131 = call "Ref_Num_XYGraph_appearance.vi"("Capacitance Results Temp Array"=w280, "Test Voltages Results Temp Array"=w281, "error in (no error)"=w279, "XY Graph NEW"=w277) -> ("error out"=w278:errorcluster)  [unwired: 7 in]
              n132 = Subtract(x=w272, y=1) -> (x-y=w271:i32)
              n133 = property class="Arr (strict)"(reference=w274) -> ("Value"=w275:dbl[][])  [unwired: 1 in, 2 out]
              n134 = Replace Array Subset(array=w275, new element=w270, index (row)=w271) -> (w276:dbl[][])  [unwired: 1 in]
              n135 = call-poly <vilib>:"Write Delimited Spreadsheet.vi"("file path (dialog if empty)"=w286, "format (%.6f)"="%.6f" ("format (%.3f)"), "1D data"=w270, "append to file? (new file:F)"=TRUE, "error in (no error)"=w278, "delimiter (\\t)"="," ("delimiter (\\t)")) -> ("error out"=w294:errorcluster)  [unwired: 8 in, 1 out]
              n136 = case shown="No Error" w294 {
                selector: w294 -> [w307 _]
                tunnel: w284 -> [w314 _]
                tunnel: w272 -> [w313 _]
                tunnel: [w312 _] -> w296
                tunnel: w285 -> [w311 _]
                tunnel: [w310 _] -> w293
                frame No Error {
                  n137 = flat-sequence {
                    tunnel: w314 -> [w320]
                    tunnel: w311 -> [w318]
                    tunnel: [w315] -> w308
                    tunnel: w307 -> [w315]
                    tunnel: [w321] -> w309
                    tunnel: w308 -> [w321]
                    tunnel: w313 -> [w325]
                    tunnel: [w324] -> w312
                    tunnel: [w323] -> w310
                    tunnel: w309 -> [w323]
                    frame #0 {
                      n138 = local write "Status : Running+-"(FALSE ("Status : Running+-")) -> ()
                      n139 = property class="Bool (strict)"(reference=w318, "Value"=FALSE) -> ()  [unwired: 1 in, 2 out]
                      n140 = property class="Bool (strict)"(reference=w320, "Value"=FALSE) -> ()  [unwired: 1 in, 2 out]
                    }
                    frame #1 {
                      n141 = Wait (ms)(milliseconds to wait=u32 350) -> ()  [unwired: 1 out]
                    }
                    frame #2 {
                      n142 = Increment(x=w325) -> (x+1=w324:i32)
                    }
                  }
                }
                frame Error {
                }
              }
              n143 = property class="Arr (strict)"(reference=w274, "Value"=w276) -> ()  [unwired: 1 in, 2 out]
              n144 = Wait (ms)(milliseconds to wait=u32 800) -> ()  [unwired: 1 out]
            }
          }
        }
        n145 = property class="DigNum (strict)"(reference=w238, "Value"=w239) -> ()  [unwired: 1 in, 2 out]
      }
    }
    n146 = property class="Bool (strict)"(reference=w209) -> ("Value"=w208:bool)  [unwired: 1 in, 2 out]
  }
  n147 = local write "error out"(w38) -> ()
